vi "Set Target Groups.vi"(8 "error in (no error)":errorcluster, 10 "Target Groups":map{string, T1}(c390), 11 "Node Config in":refnum<class "Node Config.lvclass">) -> (0 "error out":errorcluster, 3 "Node Config out":refnum<class "Node Config.lvclass">)   [LabVIEW 2020, in "VectoConfig.lvlib" / "Node Config.lvclass"]
uses:
  Node Config.lvclass
  Node Config.lvclass/Node Config.ctl
  VectoConfig/Target Group Info.ctl
  VectoConfig/VectoConfig.lvlib
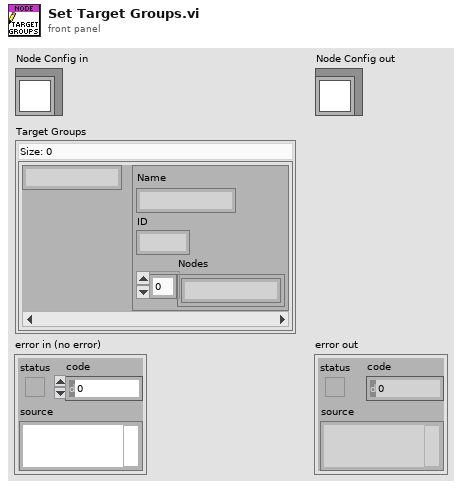
[diagram p1: front panel]
types:
  T1 = typedef "VectoConfig.lvlib/Target Group Info.ctl" = cluster{"Name":string, "ID":u32, "Nodes":string[]}
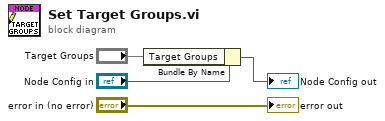
[diagram p0: block diagram]
diagram:
  n1 = Bundle By Name(cluster="Node Config in", "Target Groups"="Target Groups") -> (→"Node Config out":refnum<class "Node Config.lvclass">)
  "error out" <- "error in (no error)"
